vi "Time difference in minutes.vi"(10 "Start time":timestamp, 11 "Current time":timestamp) -> (3 "Difference (min)":i64)   [LabVIEW 2015]
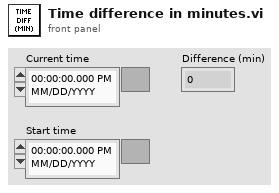
[diagram p1: front panel]
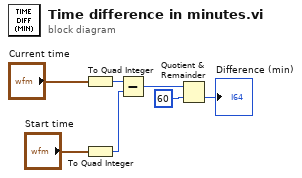
[diagram p0: block diagram]
diagram:
  n1 = To Quad Integer(1:"Current time") -> (0:w3:i64)
  n2 = To Quad Integer(1:"Start time") -> (0:w4:i64)
  n3 = Subtract(x=w3, y=w4) -> (x-y=w5:i64)
  n4 = Quotient & Remainder(x=w5, y=i64 60) -> (floor(x/y)=→"Difference (min)":i64)  [unwired: 1 out]
